vi "Auth Method.vi"(11 "TicketAuthentactor in":refnum<class "TicketAuthentactor.lvclass">) -> (2 "Authmethod":string, 3 "TicketAuthentactor out":refnum<class "TicketAuthentactor.lvclass">)   [LabVIEW 2020, in "wamplv.lvlib" / "TicketAuthentactor.lvclass"]
uses:
  TicketAuthentactor.lvclass
  TicketAuthentactor.lvclass/TicketAuthentactor.ctl
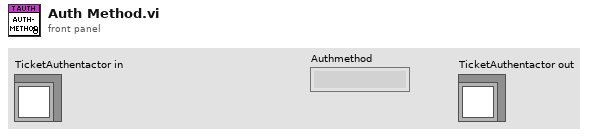
[diagram p1: front panel]
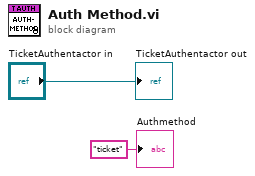
[diagram p0: block diagram]
diagram:
  "TicketAuthentactor out" <- "TicketAuthentactor in"
  "Authmethod" <- "ticket" ("Authmethod")
